vi "formulastringmaker.vi"(11 "GAUSSIAN CLUSTER":T2) -> (2 "initial parameters":dbl[](array[numeric]), 3 "output model":T1)   [LabVIEW 2020]
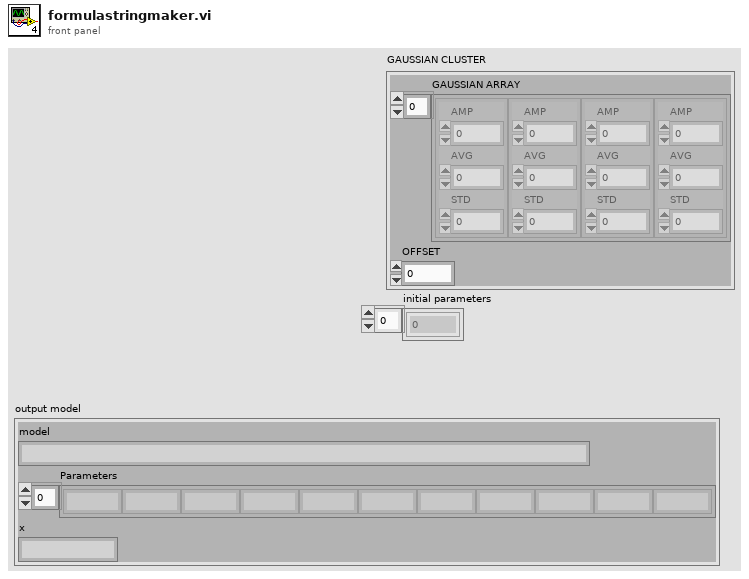
[diagram p1: front panel]
types:
  T1 = cluster{"model":string, "Parameters":string[], "x":string}
  T2 = cluster{"GAUSSIAN ARRAY":cluster{"AMP":dbl, "AVG":dbl, "STD":dbl}[], "OFFSET":dbl}
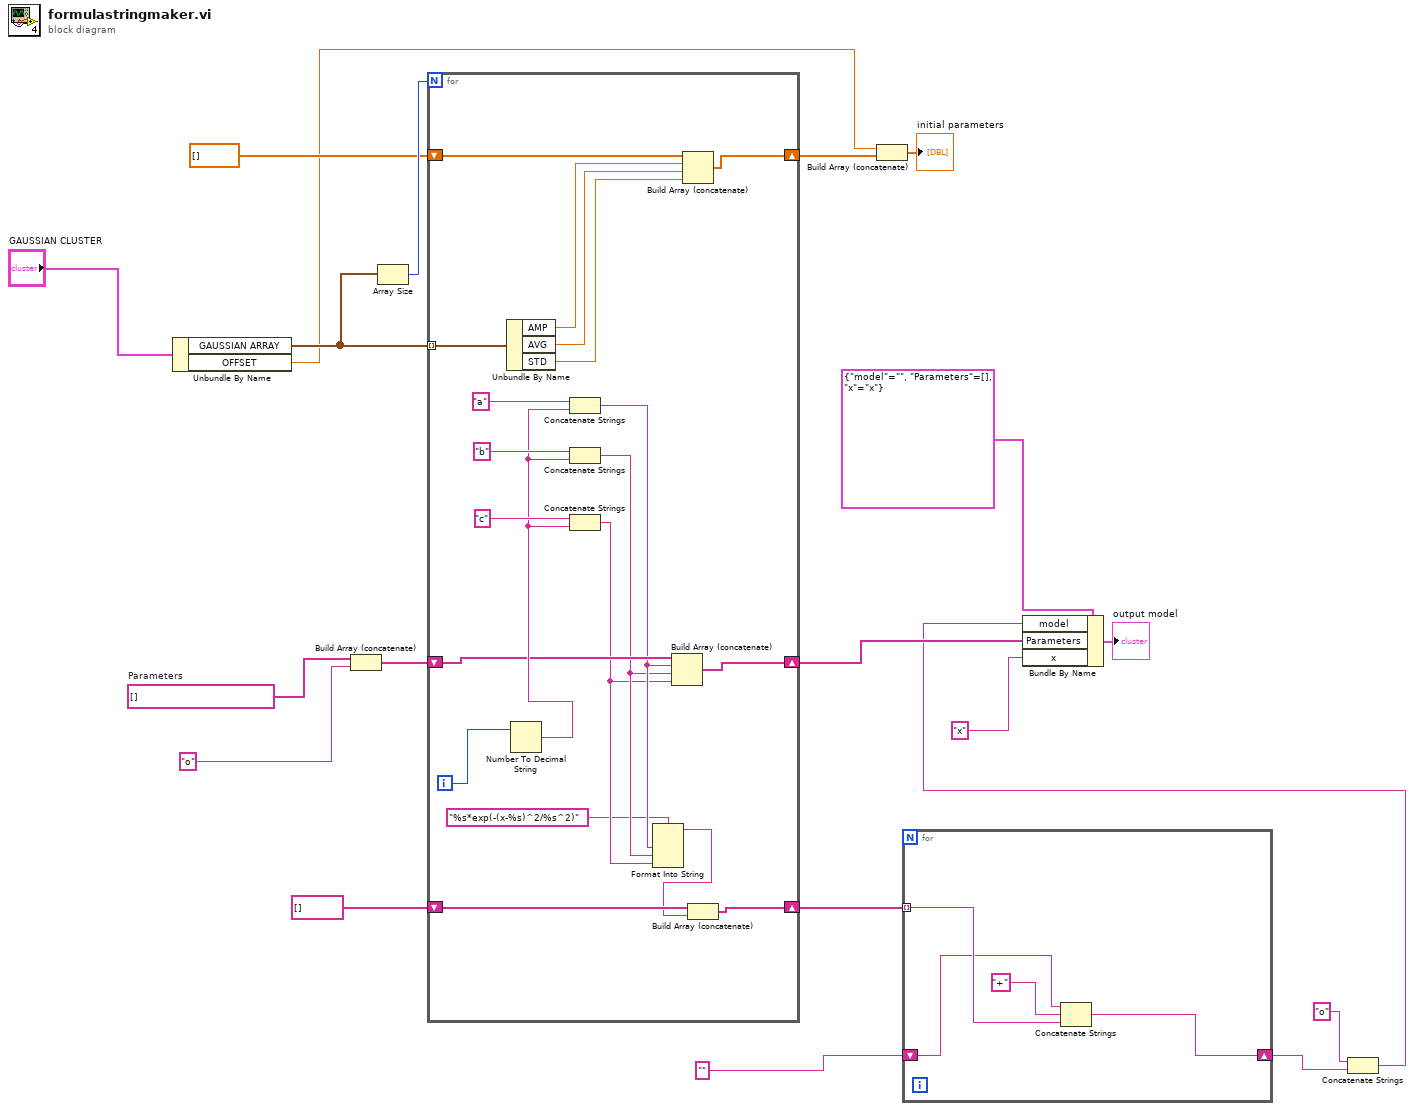
[diagram p0: block diagram]
diagram:
  w19 = string[] []  # Parameters
  n1 = Unbundle By Name("GAUSSIAN CLUSTER") -> ("GAUSSIAN ARRAY"=w5:cluster{"AMP":dbl, "AVG":dbl, "STD":dbl}[], "OFFSET"=w3:dbl)
  n2 = Build Array (concatenate)(w19, "o") -> (w17:string[])
  n3 = Array Size(array=w5) -> (size(s)=w18:i32)
  n4 = for {
    N: w18 -> [_]
    shift-right: [w34] -> w13
    shift-left: w17 -> [w35]
    shift-right: [w29] -> w12
    shift-left: string[] [] -> [w28]
    tunnel: w5 -> [w24] mode=indexing
    shift-right: [w25] -> w2
    shift-left: dbl[] [] -> [w26]
    i -> [w39]
    n5 = Unbundle By Name(w24) -> ("AMP"=w23:dbl, "AVG"=w22:dbl, "STD"=w21:dbl)
    n6 = Number To Decimal String(number=w39) -> (decimal integer string=w36:string)  [unwired: 1 in]
    n7 = Concatenate Strings("a", w36) -> (w33:string)
    n8 = Concatenate Strings("b", w36) -> (w32:string)
    n9 = Concatenate Strings("c", w36) -> (w31:string)
    n10 = Format Into String(format string="%s*exp(-(x-%s)^2/%s^2)", w33, w32, w31) -> (resulting string=w27:string)  [unwired: 2 in, 1 out]
    n11 = Build Array (concatenate)(w35, w33, w32, w31) -> (w34:string[])
    n12 = Build Array (concatenate)(w26, w23, w22, w21) -> (w25:dbl[])
    n13 = Build Array (concatenate)(w28, w27) -> (w29:string[])
  }
  n14 = Build Array (concatenate)(w3, w2) -> (→"initial parameters":dbl[])
  n15 = for {
    tunnel: w12 -> [w43] mode=indexing
    shift-right: [w41] -> w8
    shift-left: "" -> [w42]
    n16 = Concatenate Strings(w42, "+" ("string"), w43) -> (w41:string)
  }
  n17 = Concatenate Strings("o" ("string"), w8) -> (w6:string)
  n18 = Bundle By Name(cluster=T1 {"model"="", "Parameters"=[], "x"="x"} ("model description"), "model"=w6, "Parameters"=w13, "x"="x") -> (→"output model":T1)
